vi "mav_msg_decode.vi"(0 "mav_connection_in":T11, 1 "mav_msg":T25, 3 "error in":errorcluster) -> (7 "mav_connection_out":T10, 10 "error out":errorcluster)   [LabVIEW 2023]
uses:
  pfd/pfd_global.vi
  mfd/mfd_global.vi
panel:
  out "HEARTBEAT":T1
  out "WIND":T2
  out "SCALED_PRESSURE2":T3
  out "SCALED_IMU3":T4
  out "SCALED_IMU2":T4
  out "MEMINFO":T5
  out "LOCAL_POSITION_NED":T6
  out "EKF_STATUS_REPORT":T7
  out "AHRS2":T8
  out "BATTERY_STATUS":T9
  out "AUTOPILOT_VERSION":T12
  out "VIBRATION":T13
  out "AOA_SSA":cluster{"time_usec":u64, "AOA":sgl, "SSA":sgl}
  out "AHRS3":T14
  out "AHRS":T15
  out "TERRAIN_REPORT":T16
  out "POWER_STATUS":T17
  out "TIMESYNC":T18
  out "STATUSTEXT":T19(array[cluster])
  out "POSITION_TARGET_GLOBAL_INT":T20
  out "PARAM_VALUE":T21
  out "VFR_HUD":T22
  out "RC_CHANNELS":T23
  out "MISSION_CURRENT":T24
  out "NAV_CONTROLLER_OUTPUT":T26
  out "SERVO_OUTPUT_RAW":T27
  out "GLOBAL_POSITION_INT":T28
  out "ATTITUDE":T29
  out "SCALED_PRESSURE":T3
  out "RAW_IMU":T30
  out "GPS_RAW_INT":T31
  out "SYSTEM_TIME":T32
  out "SYS_STATUS":T33
  out "Message":u32[](array[numeric])
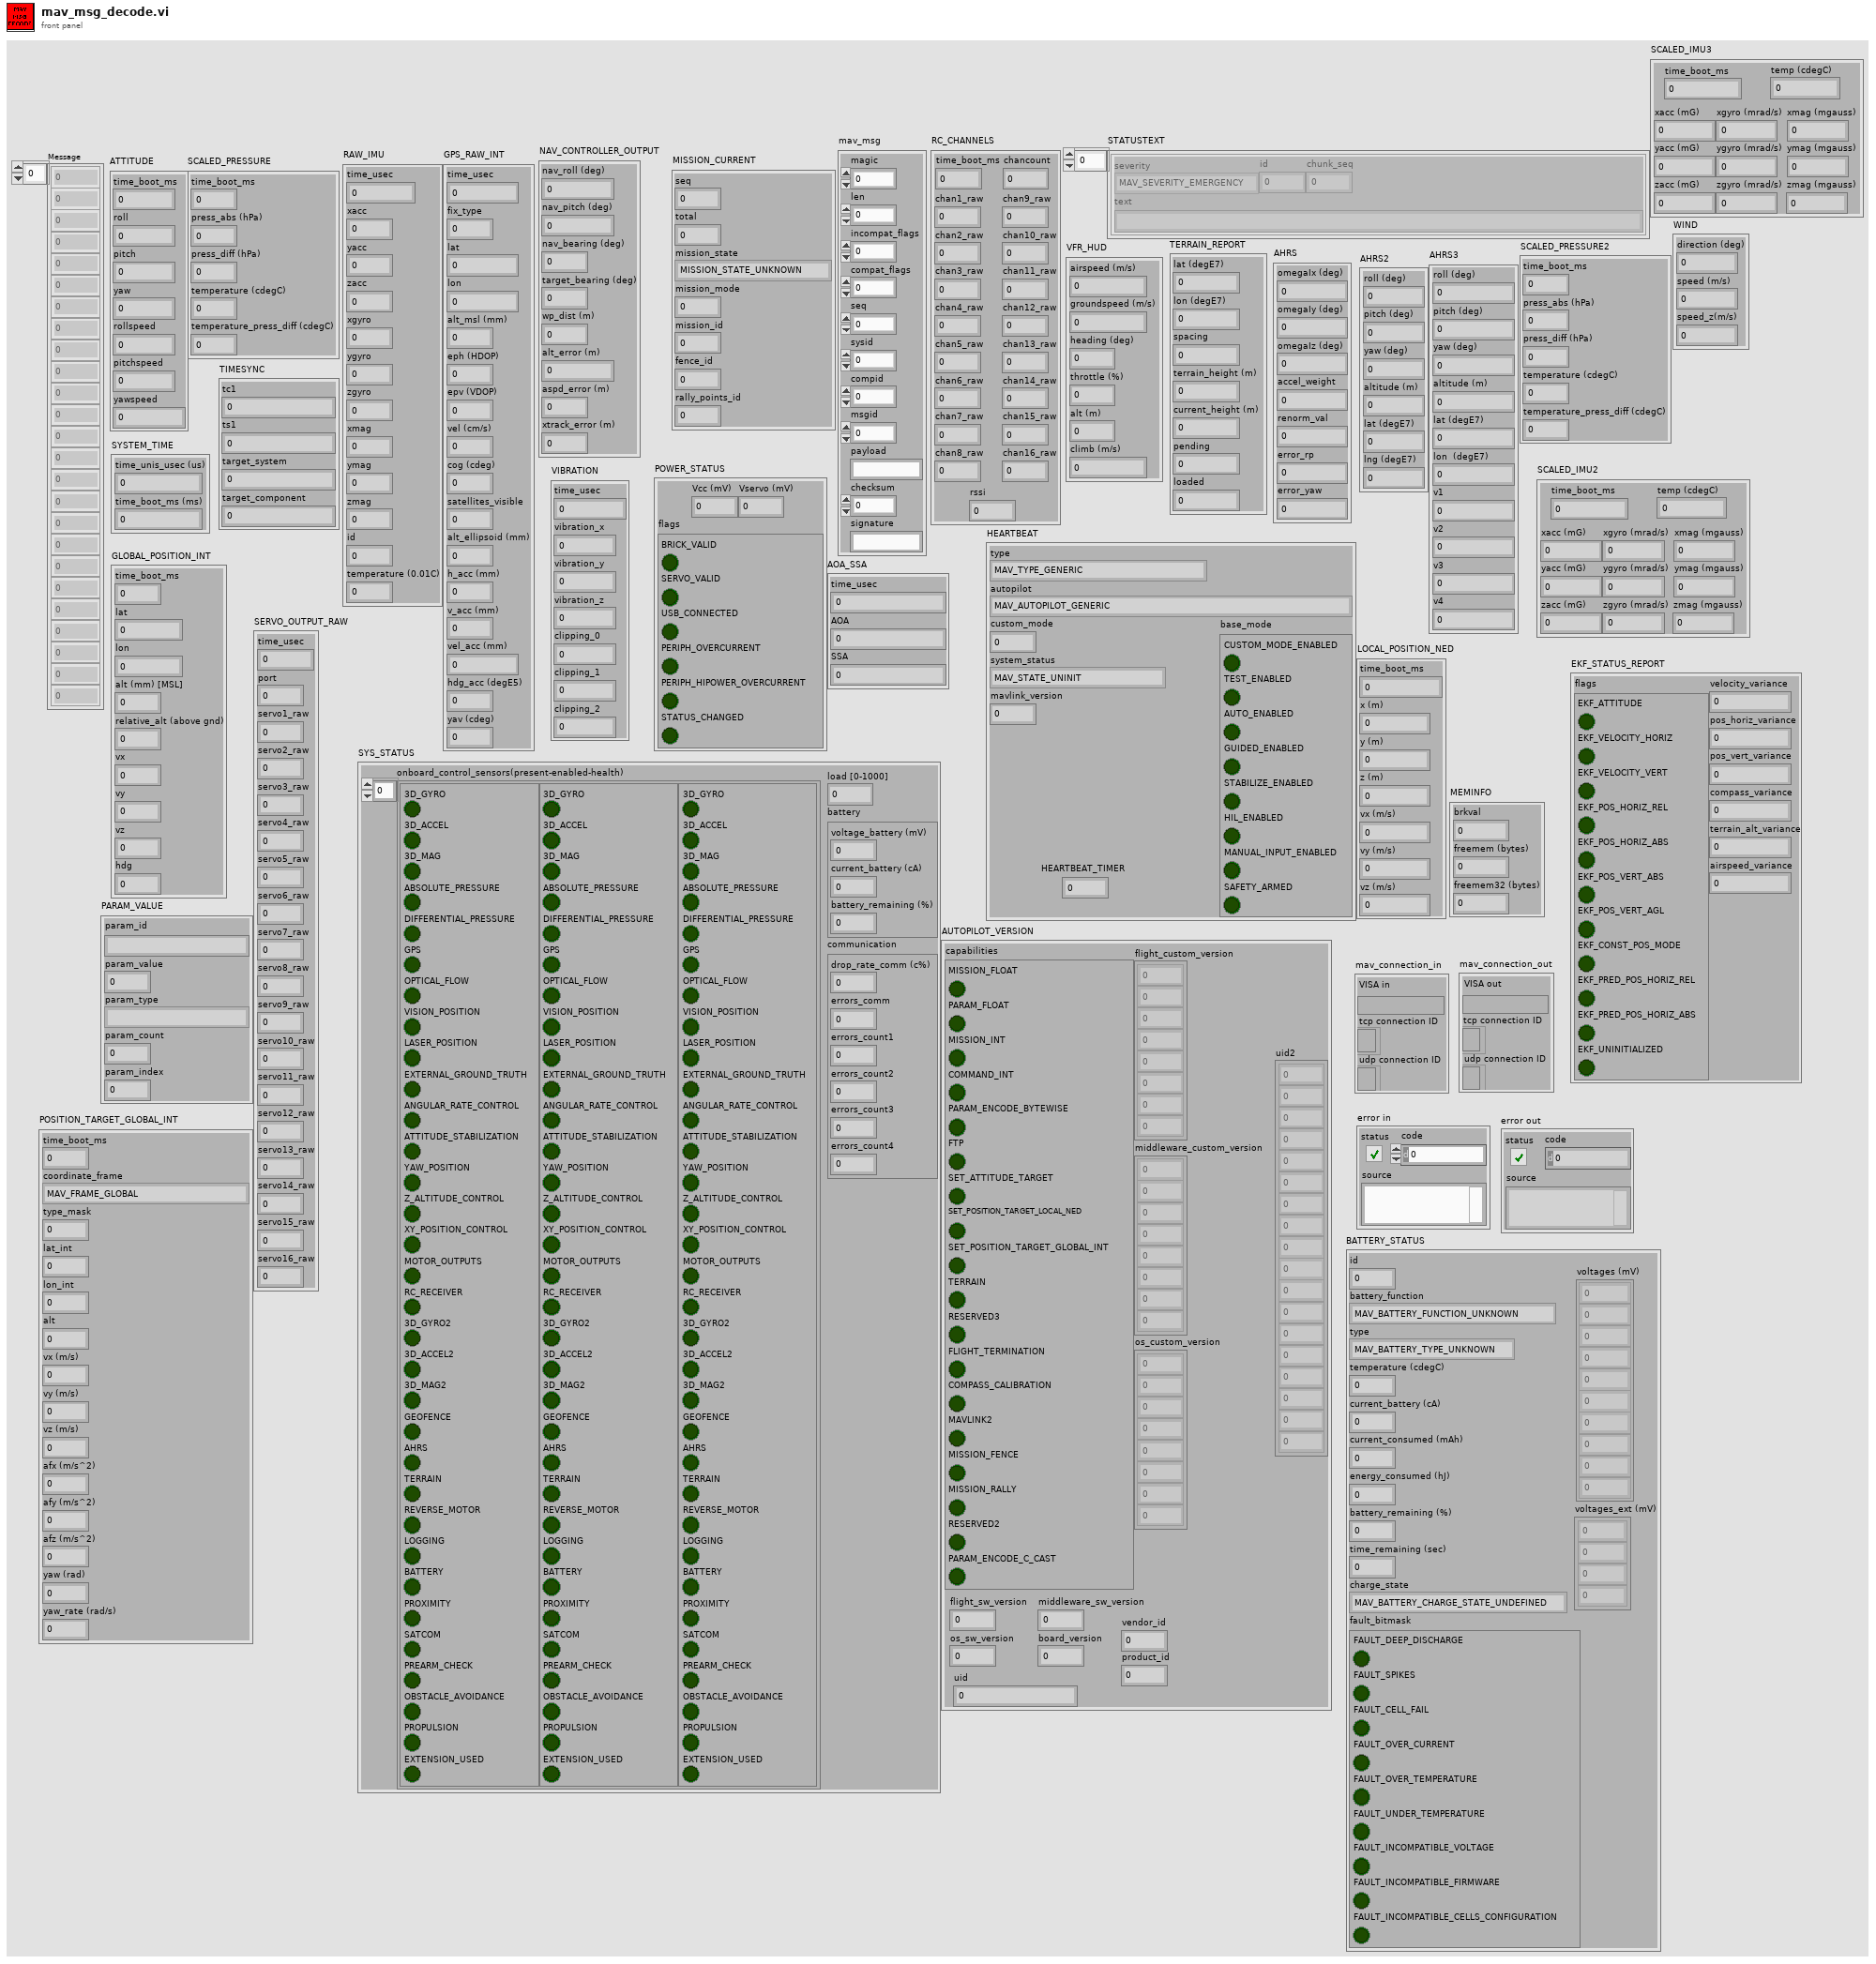
[diagram p1: front panel]
types:
  T1 = cluster{"type":enum8{"MAV_TYPE_GENERIC", "MAV_TYPE_FIXED_WING", "MAV_TYPE_QUADROTOR", "MAV_TYPE_COAXIAL", "MAV_TYPE_HELICOPTER", "MAV_TYPE_ANTENNA_TRACKER", "MAV_TYPE_GCS", "MAV_TYPE_AIRSHIP", "MAV_TYPE_FREE_BALLOON", "MAV_TYPE_ROCKET", "MAV_TYPE_GROUND_ROVER", "MAV_TYPE_SURFACE_BOAT", "MAV_TYPE_SUBMARINE", "MAV_TYPE_HEXAROTOR", "MAV_TYPE_OCTOROTOR", "MAV_TYPE_TRICOPTER", "MAV_TYPE_FLAPPING_WING", "MAV_TYPE_KITE", "MAV_TYPE_ONBOARD_CONTROLLER", "MAV_TYPE_VTOL_TAILSITTER_DUOROTOR", "MAV_TYPE_VTOL_TAILSITTER_QUADROTOR", "MAV_TYPE_VTOL_TILTROTOR", "MAV_TYPE_VTOL_FIXEDROTOR", "MAV_TYPE_VTOL_TAILSITTER", "MAV_TYPE_VTOL_TILTWING", "MAV_TYPE_VTOL_RESERVED5", "MAV_TYPE_GIMBAL", "MAV_TYPE_ADSB", "MAV_TYPE_PARAFOIL", "MAV_TYPE_DODECAROTOR", "MAV_TYPE_CAMERA", "MAV_TYPE_CHARGING_STATION", "MAV_TYPE_FLARM", "MAV_TYPE_SERVO", "MAV_TYPE_ODID", "MAV_TYPE_DECAROTOR", "MAV_TYPE_BATTERY", "MAV_TYPE_PARACHUTE", "MAV_TYPE_LOG", "MAV_TYPE_OSD", "MAV_TYPE_IMU", "MAV_TYPE_GPS", "MAV_TYPE_WINCH", "MAV_TYPE_GENERIC_MULTIROTOR", "MAV_TYPE_ILLUMINATOR"}, "autopilot":enum8{"MAV_AUTOPILOT_GENERIC", "MAV_AUTOPILOT_RESERVED", "MAV_AUTOPILOT_SLUGS", "MAV_AUTOPILOT_ARDUPILOTMEGA", "MAV_AUTOPILOT_OPENPILOT", "MAV_AUTOPILOT_GENERIC_WAYPOINTS_ONLY", "MAV_AUTOPILOT_GENERIC_WAYPOINTS_AND_SIMPLE_NAVIGATION_ONLY", "MAV_AUTOPILOT_GENERIC_MISSION_FULL", "MAV_AUTOPILOT_INVALID", "MAV_AUTOPILOT_PPZ", "MAV_AUTOPILOT_UDB", "MAV_AUTOPILOT_FP", "MAV_AUTOPILOT_PX4", "MAV_AUTOPILOT_SMACCMPILOT", "MAV_AUTOPILOT_AUTOQUAD", "MAV_AUTOPILOT_ARMAZILA", "MAV_AUTOPILOT_AEROB", "MAV_AUTOPILOT_ASLUAV", "MAV_AUTOPILOT_SMARTAP", "MAV_AUTOPILOT_AIRRAILS", "MAV_AUTOPILOT_REFLEX"}, "custom_mode":u32, "system_status":enum16{"MAV_STATE_UNINIT", "MAV_STATE_BOOT", "MAV_STATE_CALIBRATING", "MAV_STATE_STANDBY", "MAV_STATE_ACTIVE", "MAV_STATE_CRITICAL", "MAV_STATE_EMERGENCY", "MAV_STATE_POWEROFF", "MAV_STATE_FLIGHT_TERMINATION"}, "mavlink_version":u8, "base_mode":cluster{"CUSTOM_MODE_ENABLED":bool, "TEST_ENABLED":bool, "AUTO_ENABLED":bool, "GUIDED_ENABLED":bool, "STABILIZE_ENABLED":bool, "HIL_ENABLED":bool, "MANUAL_INPUT_ENABLED":bool, "SAFETY_ARMED":bool}, "HEARTBEAT_TIMER":u32}
  T2 = cluster{"direction (deg)":sgl, "speed (m/s)":sgl, "speed_z(m/s)":sgl}
  T3 = cluster{"time_boot_ms":u32, "press_abs (hPa)":sgl, "press_diff (hPa)":sgl, "temperature (cdegC)":i16, "temperature_press_diff (cdegC)":i16}
  T4 = cluster{"time_boot_ms":u32, "xacc (mG)":i16, "yacc (mG)":i16, "zacc (mG)":i16, "xgyro (mrad/s)":i16, "ygyro (mrad/s)":i16, "zgyro (mrad/s)":i16, "xmag (mgauss)":i16, "ymag (mgauss)":i16, "zmag (mgauss)":i16, "temp (cdegC)":i16}
  T5 = cluster{"brkval":u16, "freemem (bytes)":u16, "freemem32 (bytes)":u32}
  T6 = cluster{"time_boot_ms":u32, "x (m)":sgl, "y (m)":sgl, "z (m)":sgl, "vx (m/s)":sgl, "vy (m/s)":sgl, "vz (m/s)":sgl}
  T7 = cluster{"flags":cluster{"EKF_ATTITUDE":bool, "EKF_VELOCITY_HORIZ":bool, "EKF_VELOCITY_VERT":bool, "EKF_POS_HORIZ_REL":bool, "EKF_POS_HORIZ_ABS":bool, "EKF_POS_VERT_ABS":bool, "EKF_POS_VERT_AGL":bool, "EKF_CONST_POS_MODE":bool, "EKF_PRED_POS_HORIZ_REL":bool, "EKF_PRED_POS_HORIZ_ABS":bool, "EKF_UNINITIALIZED":bool}, "velocity_variance":sgl, "pos_horiz_variance":sgl, "pos_vert_variance":sgl, "compass_variance":sgl, "terrain_alt_variance":sgl, "airspeed_variance":sgl}
  T8 = cluster{"roll (deg)":sgl, "pitch (deg)":sgl, "yaw (deg)":sgl, "altitude (m)":sgl, "lat (degE7)":i32, "lng (degE7)":i32}
  T9 = cluster{"id":u8, "battery_function":enum8{"MAV_BATTERY_FUNCTION_UNKNOWN", "MAV_BATTERY_FUNCTION_ALL", "MAV_BATTERY_FUNCTION_PROPULSION", "MAV_BATTERY_FUNCTION_AVIONICS", "MAV_BATTERY_FUNCTION_PAYLOAD"}, "type":enum8{"MAV_BATTERY_TYPE_UNKNOWN", "MAV_BATTERY_TYPE_LIPO", "MAV_BATTERY_TYPE_LIFE", "MAV_BATTERY_TYPE_LION", "MAV_BATTERY_TYPE_NIMH"}, "temperature (cdegC)":i16, "voltages (mV)":u16[], "current_battery (cA)":i16, "current_consumed (mAh)":i32, "energy_consumed (hJ)":i32, "battery_remaining (%)":i8, "time_remaining (sec)":i32, "charge_state":enum8{"MAV_BATTERY_CHARGE_STATE_UNDEFINED", "MAV_BATTERY_CHARGE_STATE_OK", "MAV_BATTERY_CHARGE_STATE_LOW", "MAV_BATTERY_CHARGE_STATE_CRITICAL", "MAV_BATTERY_CHARGE_STATE_EMERGENCY", "MAV_BATTERY_CHARGE_STATE_FAILED", "MAV_BATTERY_CHARGE_STATE_UNHEALTHY", "MAV_BATTERY_CHARGE_STATE_CHARGING"}, "voltages_ext (mV)":u16[], "fault_bitmask":cluster{"FAULT_DEEP_DISCHARGE":bool, "FAULT_SPIKES":bool, "FAULT_CELL_FAIL":bool, "FAULT_OVER_CURRENT":bool, "FAULT_OVER_TEMPERATURE":bool, "FAULT_UNDER_TEMPERATURE":bool, "FAULT_INCOMPATIBLE_VOLTAGE":bool, "FAULT_INCOMPATIBLE_FIRMWARE":bool, "FAULT_INCOMPATIBLE_CELLS_CONFIGURATION":bool}}
  T10 = cluster{"VISA out":refnum<visa-resource-name>, "tcp connection ID":refnum<k5>, "udp connection ID":refnum<k16>}
  T11 = cluster{"VISA in":refnum<visa-resource-name>, "tcp connection ID":refnum<k5>, "udp connection ID":refnum<k16>}
  T12 = cluster{"flight_sw_version":u32, "middleware_sw_version":u32, "os_sw_version":u32, "board_version":u32, "capabilities":cluster{"MISSION_FLOAT":bool, "PARAM_FLOAT":bool, "MISSION_INT":bool, "COMMAND_INT":bool, "PARAM_ENCODE_BYTEWISE":bool, "FTP":bool, "SET_ATTITUDE_TARGET":bool, "SET_POSITION_TARGET_LOCAL_NED":bool, "SET_POSITION_TARGET_GLOBAL_INT":bool, "TERRAIN":bool, "RESERVED3":bool, "FLIGHT_TERMINATION":bool, "COMPASS_CALIBRATION":bool, "MAVLINK2":bool, "MISSION_FENCE":bool, "MISSION_RALLY":bool, "RESERVED2":bool, "PARAM_ENCODE_C_CAST":bool}, "flight_custom_version":u8[], "middleware_custom_version":u8[], "os_custom_version":u8[], "vendor_id":u16, "product_id":u16, "uid":u64, "uid2":u8[]}
  T13 = cluster{"time_usec":u64, "vibration_x":sgl, "vibration_y":sgl, "vibration_z":sgl, "clipping_0":u32, "clipping_1":u32, "clipping_2":u32}
  T14 = cluster{"roll (deg)":sgl, "pitch (deg)":sgl, "yaw (deg)":sgl, "altitude (m)":sgl, "lat (degE7)":i32, "lon  (degE7)":i32, "v1":sgl, "v2":sgl, "v3":sgl, "v4":sgl}
  T15 = cluster{"omegaIx (deg)":sgl, "omegaIy (deg)":sgl, "omegaIz (deg)":sgl, "accel_weight":sgl, "renorm_val":sgl, "error_rp":sgl, "error_yaw":sgl}
  T16 = cluster{"lat (degE7)":i32, "lon (degE7)":i32, "spacing":u16, "terrain_height (m) ":sgl, "current_height (m) ":sgl, "pending":u16, "loaded":u16}
  T17 = cluster{"Vcc (mV)":u16, "Vservo (mV)":u16, "flags":cluster{"BRICK_VALID":bool, "SERVO_VALID":bool, "USB_CONNECTED":bool, "PERIPH_OVERCURRENT":bool, "PERIPH_HIPOWER_OVERCURRENT":bool, "STATUS_CHANGED":bool}}
  T18 = cluster{"tc1":i64, "ts1":i64, "target_system":u8, "target_component":u8}
  T19 = cluster{"severity":enum8{"MAV_SEVERITY_EMERGENCY", "MAV_SEVERITY_ALERT", "MAV_SEVERITY_CRITICAL", "MAV_SEVERITY_ERROR", "MAV_SEVERITY_WARNING", "MAV_SEVERITY_NOTICE", "MAV_SEVERITY_INFO", "MAV_SEVERITY_DEBUG"}, "id":u16, "chunk_seq":u8, "text":string}[]
  T20 = cluster{"time_boot_ms":u32, "coordinate_frame":enum8{"MAV_FRAME_GLOBAL", "MAV_FRAME_LOCAL_NED", "MAV_FRAME_MISSION", "MAV_FRAME_GLOBAL_RELATIVE_ALT", "MAV_FRAME_LOCAL_ENU", "MAV_FRAME_GLOBAL_INT", "MAV_FRAME_GLOBAL_RELATIVE_ALT_INT", "MAV_FRAME_LOCAL_OFFSET_NED", "MAV_FRAME_BODY_NED", "MAV_FRAME_BODY_OFFSET_NED", "MAV_FRAME_GLOBAL_TERRAIN_ALT", "MAV_FRAME_GLOBAL_TERRAIN_ALT_INT", "MAV_FRAME_BODY_FRD", "MAV_FRAME_RESERVED_13", "MAV_FRAME_RESERVED_14", "MAV_FRAME_RESERVED_15", "MAV_FRAME_RESERVED_16", "MAV_FRAME_RESERVED_17", "MAV_FRAME_RESERVED_18", "MAV_FRAME_RESERVED_19", "MAV_FRAME_LOCAL_FRD", "MAV_FRAME_LOCAL_FLU"}, "type_mask":u16, "lat_int":i32, "lon_int":i32, "alt":sgl, "vx (m/s)":sgl, "vy (m/s)":sgl, "vz (m/s)":sgl, "afx (m/s^2)":sgl, "afy (m/s^2)":sgl, "afz (m/s^2)":sgl, "yaw (rad)":sgl, "yaw_rate (rad/s)":sgl}
  T21 = cluster{"param_id":string, "param_value":sgl, "param_type":enum16{"", "MAV_PARAM_TYPE_UINT8", "MAV_PARAM_TYPE_INT8", "MAV_PARAM_TYPE_UINT16", "MAV_PARAM_TYPE_INT16", "MAV_PARAM_TYPE_UINT32", "MAV_PARAM_TYPE_INT32", "MAV_PARAM_TYPE_UINT64", "MAV_PARAM_TYPE_INT64", "MAV_PARAM_TYPE_REAL32", "MAV_PARAM_TYPE_REAL64"}, "param_count":u16, "param_index":u16}
  T22 = cluster{"airspeed (m/s)":sgl, "groundspeed (m/s)":sgl, "heading (deg) ":i16, "throttle (%) ":u16, "alt (m)":sgl, "climb (m/s)":sgl}
  T23 = cluster{"time_boot_ms":u32, "chancount":u8, "chan1_raw":u16, "chan2_raw":u16, "chan3_raw":u16, "chan4_raw":u16, "chan5_raw":u16, "chan6_raw":u16, "chan7_raw":u16, "chan8_raw":u16, "chan9_raw":u16, "chan10_raw":u16, "chan11_raw":u16, "chan12_raw":u16, "chan13_raw":u16, "chan14_raw":u16, "chan15_raw":u16, "chan16_raw":u16, "rssi":u8}
  T24 = cluster{"seq":u16, "total":u16, "mission_state":enum8{"MISSION_STATE_UNKNOWN", "MISSION_STATE_NO_MISSION", "MISSION_STATE_NOT_STARTED", "MISSION_STATE_ACTIVE", "MISSION_STATE_PAUSED", "MISSION_STATE_COMPLETE"}, "mission_mode":u8, "mission_id":u32, "fence_id":u32, "rally_points_id":u32}
  T25 = cluster{"len":u8, "incompat_flags":u8, "compat_flags":u8, "seq":u8, "sysid":u8, "compid":u8, "msgid":u32, "magic":u8, "payload":string, "checksum":u16, "signature":string}
  T26 = cluster{"nav_roll (deg)":sgl, "nav_pitch (deg)":sgl, "nav_bearing (deg)":i16, "target_bearing (deg)":i16, "wp_dist (m)":u16, "alt_error (m)":sgl, "aspd_error (m)":sgl, "xtrack_error (m)":sgl}
  T27 = cluster{"time_usec":u32, "port":u8, "servo1_raw":u16, "servo2_raw":u16, "servo3_raw":u16, "servo4_raw":u16, "servo5_raw":u16, "servo6_raw":u16, "servo7_raw":u16, "servo8_raw":u16, "servo9_raw":u16, "servo10_raw":u16, "servo11_raw":u16, "servo12_raw":u16, "servo13_raw":u16, "servo14_raw":u16, "servo15_raw":u16, "servo16_raw":u16}
  T28 = cluster{"time_boot_ms":u32, "lat":i32, "lon":i32, "alt (mm) [MSL]":i32, "relative_alt (above gnd)":i32, "vx":i16, "vy":i16, "vz":i16, "hdg":u16}
  T29 = cluster{"time_boot_ms":u32, "roll":sgl, "pitch":sgl, "yaw":sgl, "rollspeed":sgl, "pitchspeed":sgl, "yawspeed":sgl}
  T30 = cluster{"time_usec":u64, "xacc":i16, "yacc":i16, "zacc":i16, "xgyro":i16, "ygyro":i16, "zgyro":i16, "xmag":i16, "ymag":i16, "zmag":i16, "id":u8, "temperature (0.01C)":i16}
  T31 = cluster{"time_usec":u64, "fix_type":u8, "lat":i32, "lon":i32, "alt_msl (mm)":i32, "eph (HDOP)":u16, "epv (VDOP)":u16, "vel (cm/s)":u16, "cog (cdeg)":u16, "satellites_visible":u8, "alt_ellipsoid (mm)":i32, "h_acc (mm)":u32, "v_acc (mm)":u32, "vel_acc (mm)":u32, "hdg_acc (degE5)":u32, "yav (cdeg)":u16}
  T32 = cluster{"time_unis_usec (us)":u64, "time_boot_ms (ms)":u32}
  T33 = cluster{"onboard_control_sensors(present-enabled-health)":cluster{"3D_GYRO":bool, "3D_ACCEL":bool, "3D_MAG":bool, "ABSOLUTE_PRESSURE":bool, "DIFFERENTIAL_PRESSURE":bool, "GPS":bool, "OPTICAL_FLOW":bool, "VISION_POSITION":bool, "LASER_POSITION":bool, "EXTERNAL_GROUND_TRUTH":bool, "ANGULAR_RATE_CONTROL":bool, "ATTITUDE_STABILIZATION":bool, "YAW_POSITION":bool, "Z_ALTITUDE_CONTROL":bool, "XY_POSITION_CONTROL":bool, "MOTOR_OUTPUTS":bool, "RC_RECEIVER":bool, "3D_GYRO2":bool, "3D_ACCEL2":bool, "3D_MAG2":bool, "GEOFENCE":bool, "AHRS":bool, "TERRAIN":bool, "REVERSE_MOTOR":bool, "LOGGING":bool, "BATTERY":bool, "PROXIMITY":bool, "SATCOM":bool, "PREARM_CHECK":bool, "OBSTACLE_AVOIDANCE":bool, "PROPULSION":bool, "EXTENSION_USED":bool}[], "load [0-1000]":u16, "battery":cluster{"voltage_battery (mV)":u16, "current_battery (cA)":i16, "battery_remaining (%)":i8}, "communication":cluster{"drop_rate_comm (c%)":u16, "errors_comm":u16, "errors_count1":u16, "errors_count2":u16, "errors_count3":u16, "errors_count4":u16}}
  T34 = cluster{"chancount":u8, "chan1_raw":u16, "chan2_raw":u16, "chan3_raw":u16, "chan4_raw":u16, "chan5_raw":u16, "chan6_raw":u16, "chan7_raw":u16, "chan8_raw":u16, "chan9_raw":u16, "chan10_raw":u16, "chan11_raw":u16, "chan12_raw":u16, "chan13_raw":u16, "chan14_raw":u16, "chan15_raw":u16, "chan16_raw":u16, "rssi":u8}
  T35 = cluster{"HEARTBEAT":cluster{"type":enum8{"MAV_TYPE_GENERIC", "MAV_TYPE_FIXED_WING", "MAV_TYPE_QUADROTOR", "MAV_TYPE_COAXIAL", "MAV_TYPE_HELICOPTER", "MAV_TYPE_ANTENNA_TRACKER", "MAV_TYPE_GCS", "MAV_TYPE_AIRSHIP", "MAV_TYPE_FREE_BALLOON", "MAV_TYPE_ROCKET", "MAV_TYPE_GROUND_ROVER", "MAV_TYPE_SURFACE_BOAT", "MAV_TYPE_SUBMARINE", "MAV_TYPE_HEXAROTOR", "MAV_TYPE_OCTOROTOR", "MAV_TYPE_TRICOPTER", "MAV_TYPE_FLAPPING_WING", "MAV_TYPE_KITE", "MAV_TYPE_ONBOARD_CONTROLLER", "MAV_TYPE_VTOL_TAILSITTER_DUOROTOR", "MAV_TYPE_VTOL_TAILSITTER_QUADROTOR", "MAV_TYPE_VTOL_TILTROTOR", "MAV_TYPE_VTOL_FIXEDROTOR", "MAV_TYPE_VTOL_TAILSITTER", "MAV_TYPE_VTOL_TILTWING", "MAV_TYPE_VTOL_RESERVED5", "MAV_TYPE_GIMBAL", "MAV_TYPE_ADSB", "MAV_TYPE_PARAFOIL", "MAV_TYPE_DODECAROTOR", "MAV_TYPE_CAMERA", "MAV_TYPE_CHARGING_STATION", "MAV_TYPE_FLARM", "MAV_TYPE_SERVO", "MAV_TYPE_ODID", "MAV_TYPE_DECAROTOR", "MAV_TYPE_BATTERY", "MAV_TYPE_PARACHUTE", "MAV_TYPE_LOG", "MAV_TYPE_OSD", "MAV_TYPE_IMU", "MAV_TYPE_GPS", "MAV_TYPE_WINCH", "MAV_TYPE_GENERIC_MULTIROTOR", "MAV_TYPE_ILLUMINATOR"}, "autopilot":enum8{"MAV_AUTOPILOT_GENERIC", "MAV_AUTOPILOT_RESERVED", "MAV_AUTOPILOT_SLUGS", "MAV_AUTOPILOT_ARDUPILOTMEGA", "MAV_AUTOPILOT_OPENPILOT", "MAV_AUTOPILOT_GENERIC_WAYPOINTS_ONLY", "MAV_AUTOPILOT_GENERIC_WAYPOINTS_AND_SIMPLE_NAVIGATION_ONLY", "MAV_AUTOPILOT_GENERIC_MISSION_FULL", "MAV_AUTOPILOT_INVALID", "MAV_AUTOPILOT_PPZ", "MAV_AUTOPILOT_UDB", "MAV_AUTOPILOT_FP", "MAV_AUTOPILOT_PX4", "MAV_AUTOPILOT_SMACCMPILOT", "MAV_AUTOPILOT_AUTOQUAD", "MAV_AUTOPILOT_ARMAZILA", "MAV_AUTOPILOT_AEROB", "MAV_AUTOPILOT_ASLUAV", "MAV_AUTOPILOT_SMARTAP", "MAV_AUTOPILOT_AIRRAILS", "MAV_AUTOPILOT_REFLEX"}, "custom_mode":u32, "system_status":enum16{"MAV_STATE_UNINIT", "MAV_STATE_BOOT", "MAV_STATE_CALIBRATING", "MAV_STATE_STANDBY", "MAV_STATE_ACTIVE", "MAV_STATE_CRITICAL", "MAV_STATE_EMERGENCY", "MAV_STATE_POWEROFF", "MAV_STATE_FLIGHT_TERMINATION"}, "mavlink_version":u8, "base_mode":cluster{"CUSTOM_MODE_ENABLED":bool, "TEST_ENABLED":bool, "AUTO_ENABLED":bool, "GUIDED_ENABLED":bool, "STABILIZE_ENABLED":bool, "HIL_ENABLED":bool, "MANUAL_INPUT_ENABLED":bool, "SAFETY_ARMED":bool}, "HEARTBEAT_TIMER":u32}, "Batt Stats":cluster{"Active":bool, "State":bool}, "Sat Stats":cluster{"Active":bool, "State":bool}, "Radio Stats":cluster{"Active":bool, "State":bool}, "Sensor Stats":cluster{"Active":bool, "State":bool}}
  T36 = cluster{"3D_GYRO":bool, "3D_ACCEL":bool, "3D_MAG":bool, "ABSOLUTE_PRESSURE":bool, "DIFFERENTIAL_PRESSURE":bool, "GPS":bool, "OPTICAL_FLOW":bool, "VISION_POSITION":bool, "LASER_POSITION":bool, "EXTERNAL_GROUND_TRUTH":bool, "ANGULAR_RATE_CONTROL":bool, "ATTITUDE_STABILIZATION":bool, "YAW_POSITION":bool, "Z_ALTITUDE_CONTROL":bool, "XY_POSITION_CONTROL":bool, "MOTOR_OUTPUTS":bool, "RC_RECEIVER":bool, "3D_GYRO2":bool, "3D_ACCEL2":bool, "3D_MAG2":bool, "GEOFENCE":bool, "AHRS":bool, "TERRAIN":bool, "REVERSE_MOTOR":bool, "LOGGING":bool, "BATTERY":bool, "PROXIMITY":bool, "SATCOM":bool, "PREARM_CHECK":bool, "OBSTACLE_AVOIDANCE":bool, "PROPULSION":bool, "EXTENSION_USED":bool}[]
  T37 = cluster{"voltage_battery (mV)":u16, "current_battery (cA)":i16, "battery_remaining (%)":i8}
  T38 = cluster{"3D_GYRO":bool, "3D_ACCEL":bool, "3D_MAG":bool, "ABSOLUTE_PRESSURE":bool, "DIFFERENTIAL_PRESSURE":bool, "GPS":bool, "OPTICAL_FLOW":bool, "VISION_POSITION":bool, "LASER_POSITION":bool, "EXTERNAL_GROUND_TRUTH":bool, "ANGULAR_RATE_CONTROL":bool, "ATTITUDE_STABILIZATION":bool, "YAW_POSITION":bool, "Z_ALTITUDE_CONTROL":bool, "XY_POSITION_CONTROL":bool, "MOTOR_OUTPUTS":bool, "RC_RECEIVER":bool, "3D_GYRO2":bool, "3D_ACCEL2":bool, "3D_MAG2":bool, "GEOFENCE":bool, "AHRS":bool, "TERRAIN":bool, "REVERSE_MOTOR":bool, "LOGGING":bool, "BATTERY":bool, "PROXIMITY":bool, "SATCOM":bool, "PREARM_CHECK":bool, "OBSTACLE_AVOIDANCE":bool, "PROPULSION":bool, "EXTENSION_USED":bool}
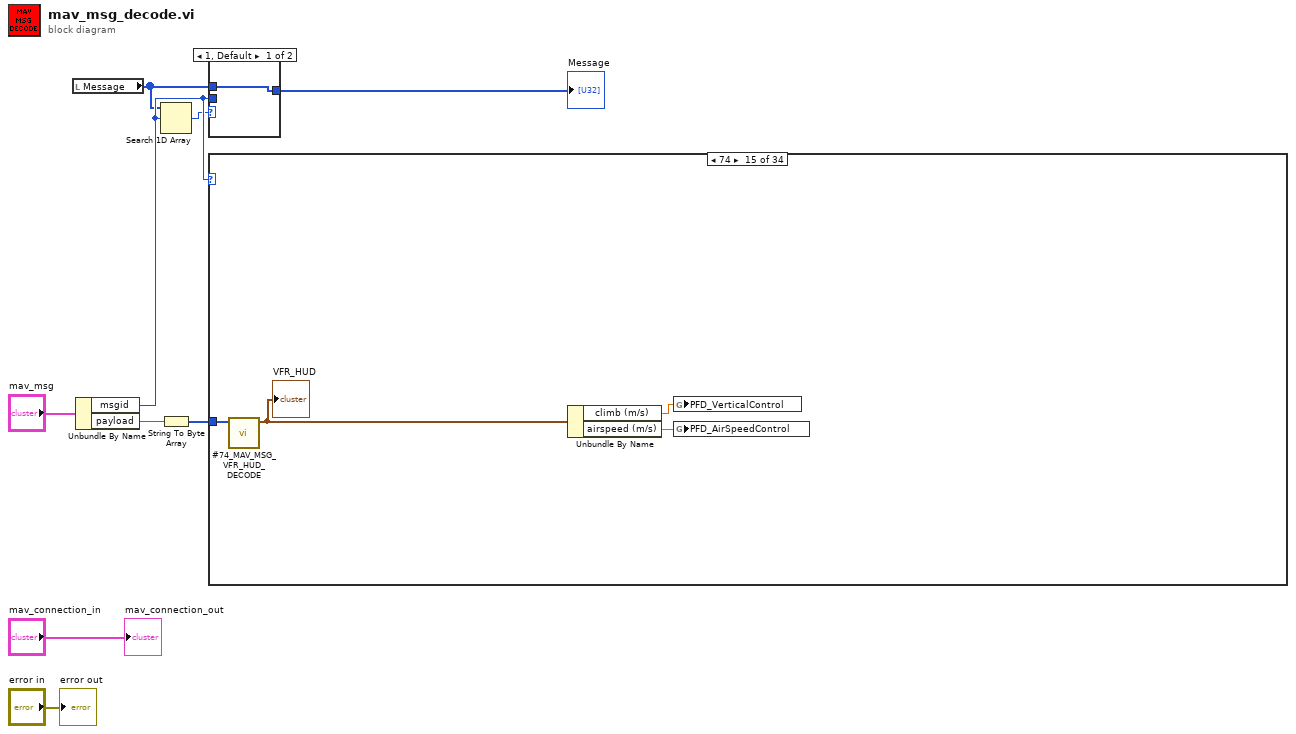
[diagram p0: block diagram]
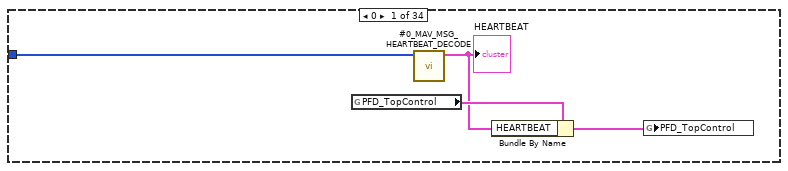
[diagram p2: hidden frame]
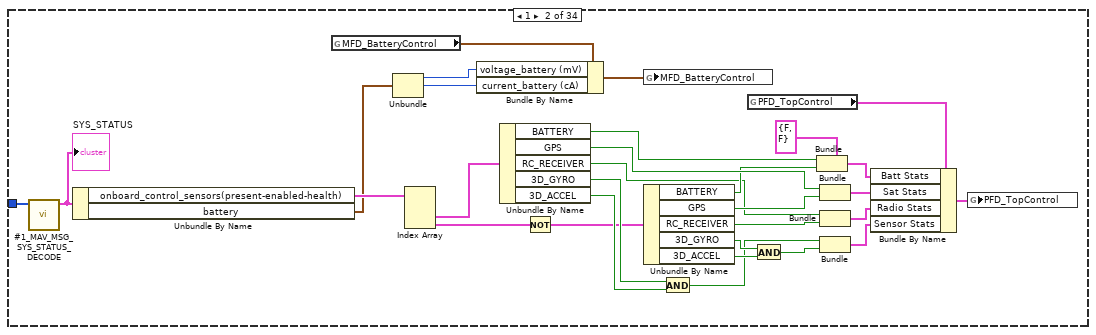
[diagram p3: hidden frame]
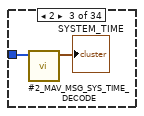
[diagram p4: hidden frame]
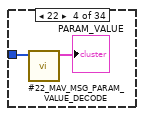
[diagram p5: hidden frame]
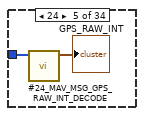
[diagram p6: hidden frame]
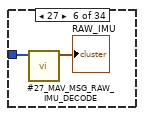
[diagram p7: hidden frame]
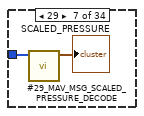
[diagram p8: hidden frame]
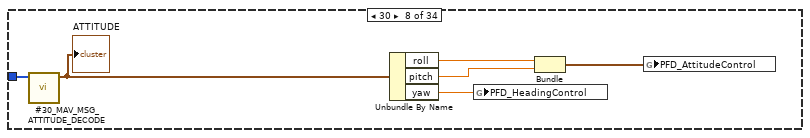
[diagram p9: hidden frame]
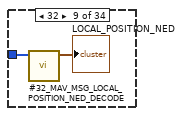
[diagram p10: hidden frame]
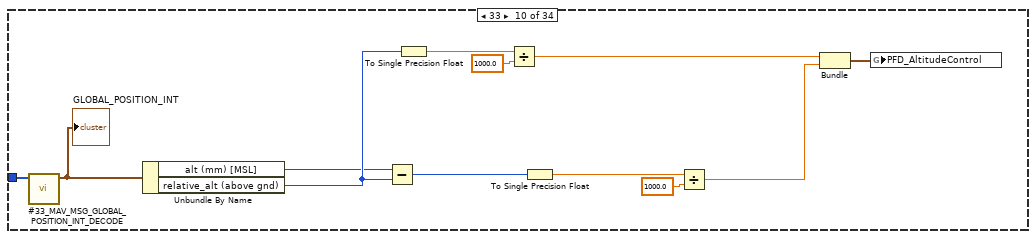
[diagram p11: hidden frame]
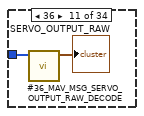
[diagram p12: hidden frame]
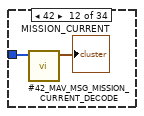
[diagram p13: hidden frame]
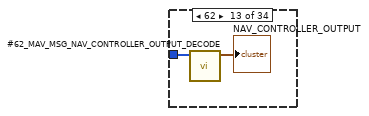
[diagram p14: hidden frame]
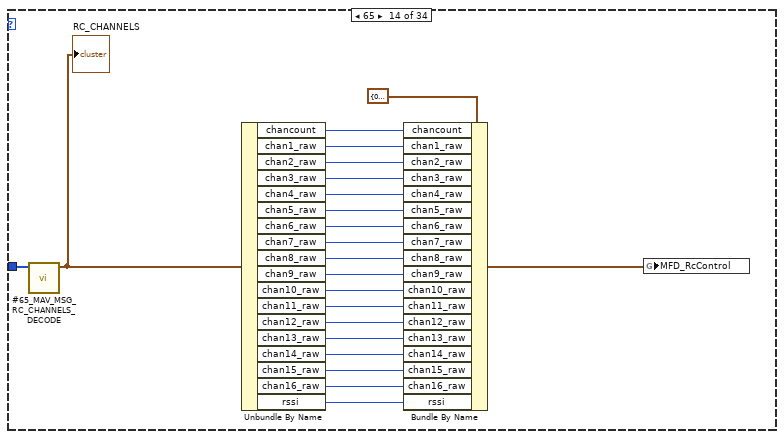
[diagram p15: hidden frame]
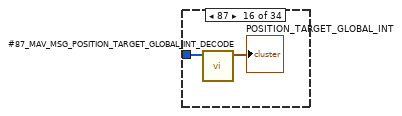
[diagram p16: hidden frame]
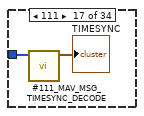
[diagram p17: hidden frame]
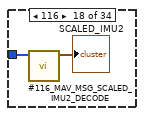
[diagram p18: hidden frame]
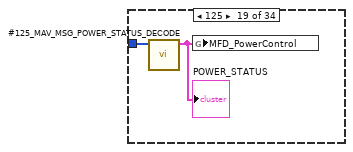
[diagram p19: hidden frame]
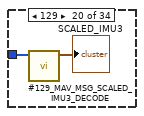
[diagram p20: hidden frame]
diagram:
  n1 = local read "Message"() -> (w3:u32[])
  n2 = Unbundle By Name("mav_msg") -> ("msgid"=w7:u32, "payload"=w8:string)
  n3 = Search 1D Array(1D array=w3, element=w7) -> (index of element=w6:i32)  [unwired: 1 in]
  n4 = String To Byte Array(string=w8) -> (unsigned byte array=w5:u8[])
  n5 = case shown="1, Default" w6 {
    tunnel: w3 -> [w10 w13]
    tunnel: [w10 w12] -> w4
    tunnel: w7 -> [_ w11]
    frame 1, Default {
    }
    frame -1 {
      n6 = Build Array (concatenate)(w13, w11) -> (w12:u32[])
    }
  }
  "Message" <- w4
  n7 = case shown="74" w7 {
    tunnel: w5 -> [w17 w47 w49 w51 w53 w55 w57 w63 w65 w77 w79 w81 w83 w105 w109 w111 w113 w115 w117 w119 w121 w123 w128 w130 w132 w134 w136 w138 w140 w142 w144 w146 _ w148]
    frame 0 {
      n8 = global read "pfd_global.vi" "PFD_TopControl"() -> (w16:T35)
      n9 = call "#0_MAV_MSG_HEARTBEAT_DECODE.vi"("mavlink_payload"=w17) -> ("HEARTBEAT"=w14:T1)  [unwired: 10 in]
      "HEARTBEAT" <- w14
      n10 = Bundle By Name(cluster=w16, "HEARTBEAT"=w14) -> (w15:T35)
      n11 = global write "pfd_global.vi" "PFD_TopControl"(w15) -> ()
    }
    frame 1 {
      n12 = call "#1_MAV_MSG_SYS_STATUS_DECODE.vi"("mavlink_payload"=w47) -> ("SYS_STATUS"=w45:T33)  [unwired: 10 in]
      "SYS_STATUS" <- w45
      n13 = Unbundle By Name(w45) -> ("onboard_control_sensors(present-enabled-health)"=w44:T36, "battery"=w22:T37)
      n14 = global read "mfd_global.vi" "MFD_BatteryControl"() -> (w21:T37)
      n15 = Unbundle(w22) -> ("voltage_battery (mV)"=w19:u16, "current_battery (cA)"=w18:i16)  [unwired: 1 out]
      n16 = Index Array(array=w44) -> (element #2=w43:T38, element #3=w24:T38)  [unwired: 3 in, 1 out]
      n17 = Bundle By Name(cluster=w21, "voltage_battery (mV)"=w19, "current_battery (cA)"=w18) -> (w20:T37)
      n18 = Unbundle By Name(w43) -> ("BATTERY"=w35:bool, "GPS"=w34:bool, "RC_RECEIVER"=w30:bool, "3D_GYRO"=w41:bool, "3D_ACCEL"=w40:bool)
      n19 = Not(x=w24) -> (.not. x?=w23:T38)
      n20 = global write "mfd_global.vi" "MFD_BatteryControl"(w20) -> ()
      n21 = Unbundle By Name(w23) -> ("BATTERY"=w32:bool, "GPS"=w33:bool, "RC_RECEIVER"=w29:bool, "3D_GYRO"=w39:bool, "3D_ACCEL"=w38:bool)
      n22 = And(x=w41, y=w40) -> (x .and. y?=w26:bool)
      n23 = global read "pfd_global.vi" "PFD_TopControl"() -> (w46:T35)
      n24 = And(x=w39, y=w38) -> (x .and. y?=w27:bool)
      n25 = Bundle(cluster=cluster{"Active":bool, "State":bool} {"Active"=FALSE, "State"=FALSE} ("Batt Stats"), "Active"=w35, "State"=w32) -> (w36:cluster{"Active":bool, "State":bool})
      n26 = Bundle("GPS"=w34, "GPS"=w33) -> (w31:cluster{"GPS":bool, "GPS":bool})  [unwired: 1 in]
      n27 = Bundle("RC_RECEIVER"=w30, "RC_RECEIVER"=w29) -> (w28:cluster{"RC_RECEIVER":bool, "RC_RECEIVER":bool})  [unwired: 1 in]
      n28 = Bundle(w26, w27) -> (w25:cluster{bool, bool})  [unwired: 1 in]
      n29 = Bundle By Name(cluster=w46, "Batt Stats"=w36, "Sat Stats"=w31, "Radio Stats"=w28, "Sensor Stats"=w25) -> (w42:T35)
      n30 = global write "pfd_global.vi" "PFD_TopControl"(w42) -> ()
    }
    frame 2 {
      n31 = call "#2_MAV_MSG_SYS_TIME_DECODE.vi"("mavlink_payload"=w49) -> ("SYSTEM_TIME"=→"SYSTEM_TIME":T32)  [unwired: 10 in]
    }
    frame 22 {
      n32 = call "#22_MAV_MSG_PARAM_VALUE_DECODE.vi"("mavlink_payload"=w51) -> ("PARAM_VALUE"=→"PARAM_VALUE":T21)  [unwired: 10 in]
    }
    frame 24 {
      n33 = call "#24_MAV_MSG_GPS_RAW_INT_DECODE.vi"("mavlink_payload"=w53) -> ("GPS_RAW_INT"=→"GPS_RAW_INT":T31)  [unwired: 10 in]
    }
    frame 27 {
      n34 = call "#27_MAV_MSG_RAW_IMU_DECODE.vi"("mavlink_payload"=w55) -> ("RAW_IMU"=→"RAW_IMU":T30)  [unwired: 10 in]
    }
    frame 29 {
      n35 = call "#29_MAV_MSG_SCALED_PRESSURE_DECODE.vi"("mavlink_payload"=w57) -> ("SCALED_PRESSURE"=→"SCALED_PRESSURE":T3)  [unwired: 10 in]
    }
    frame 30 {
      n36 = call "#30_MAV_MSG_ATTITUDE_DECODE.vi"("mavlink_payload"=w63) -> ("ATTITUDE"=w61:T29)  [unwired: 10 in]
      "ATTITUDE" <- w61
      n37 = Unbundle By Name(w61) -> ("roll"=w59:sgl, "pitch"=w60:sgl, "yaw"=w58:sgl)
      n38 = global write "pfd_global.vi" "PFD_HeadingControl"(w58) -> ()
      n39 = Bundle("roll"=w59, "pitch"=w60) -> (w62:cluster{"roll":sgl, "pitch":sgl})  [unwired: 1 in]
      n40 = global write "pfd_global.vi" "PFD_AttitudeControl"(w62) -> ()
    }
    frame 32 {
      n41 = call "#32_MAV_MSG_LOCAL_POSITION_NED_DECODE.vi"("mavlink_payload"=w65) -> ("LOCAL_POSITION_NED"=→"LOCAL_POSITION_NED":T6)  [unwired: 10 in]
    }
    frame 33 {
      n42 = call "#33_MAV_MSG_GLOBAL_POSITION_INT_DECODE.vi"("mavlink_payload"=w77) -> ("GLOBAL_POSITION_INT"=w67:T28)  [unwired: 10 in]
      "GLOBAL_POSITION_INT" <- w67
      n43 = Unbundle By Name(w67) -> ("alt (mm) [MSL]"=w70:i32, "relative_alt (above gnd)"=w71:i32)
      n44 = Subtract(x=w70, y=w71) -> (x-y=w74:i32)
      n45 = To Single Precision Float(number=w71) -> (single precision float=w72:sgl)
      n46 = Divide(x=w72, y=sgl 1000.0) -> (x/y=w73:sgl)
      n47 = To Single Precision Float(number=w74) -> (single precision float=w75:sgl)
      n48 = Divide(x=w75, y=sgl 1000.0) -> (x/y=w76:sgl)
      n49 = Bundle(w73, w76) -> (w66:cluster{sgl, sgl})  [unwired: 1 in]
      n50 = global write "pfd_global.vi" "PFD_AltitudeControl"(w66) -> ()
    }
    frame 36 {
      n51 = call "#36_MAV_MSG_SERVO_OUTPUT_RAW_DECODE.vi"("mavlink_payload"=w79) -> ("SERVO_OUTPUT_RAW"=→"SERVO_OUTPUT_RAW":T27)  [unwired: 10 in]
    }
    frame 42 {
      n52 = call "#42_MAV_MSG_MISSION_CURRENT_DECODE.vi"("mavlink_payload"=w81) -> ("MISSION_CURRENT"=→"MISSION_CURRENT":T24)  [unwired: 10 in]
    }
    frame 62 {
      n53 = call "#62_MAV_MSG_NAV_CONTROLLER_OUTPUT_DECODE.vi"("mavlink_payload"=w83) -> ("NAV_CONTROLLER_OUTPUT"=→"NAV_CONTROLLER_OUTPUT":T26)  [unwired: 10 in]
    }
    frame 65 {
      n54 = call "#65_MAV_MSG_RC_CHANNELS_DECODE.vi"("mavlink_payload"=w105) -> ("RC_CHANNELS"=w102:T23)  [unwired: 10 in]
      "RC_CHANNELS" <- w102
      n55 = Unbundle By Name(w102) -> ("chancount"=w101:u8, "chan1_raw"=w100:u16, "chan2_raw"=w99:u16, "chan3_raw"=w98:u16, "chan4_raw"=w97:u16, "chan5_raw"=w96:u16, "chan6_raw"=w95:u16, "chan7_raw"=w94:u16, "chan8_raw"=w93:u16, "chan9_raw"=w92:u16, "chan10_raw"=w91:u16, "chan11_raw"=w90:u16, "chan12_raw"=w89:u16, "chan13_raw"=w88:u16, "chan14_raw"=w87:u16, "chan15_raw"=w86:u16, "chan16_raw"=w85:u16, "rssi"=w84:u8)
      n56 = Bundle By Name(cluster=T34 {"chancount"=0, "chan1_raw"=0, "chan2_raw"=0, "chan3_raw"=0, "chan4_raw"=0, "chan5_raw"=0, "chan6_raw"=0, "chan7_raw"=0, "chan8_raw"=0, "chan9_raw"=0, "chan10_raw"=0, "chan11_raw"=0, "chan12_raw"=0, "chan13_raw"=0, "chan14_raw"=0, "chan15_raw"=0, "chan16_raw"=0, "rssi"=0} ("MFD_RcControl"), "chancount"=w101, "chan1_raw"=w100, "chan2_raw"=w99, "chan3_raw"=w98, "chan4_raw"=w97, "chan5_raw"=w96, "chan6_raw"=w95, "chan7_raw"=w94, "chan8_raw"=w93, "chan9_raw"=w92, "chan10_raw"=w91, "chan11_raw"=w90, "chan12_raw"=w89, "chan13_raw"=w88, "chan14_raw"=w87, "chan15_raw"=w86, "chan16_raw"=w85, "rssi"=w84) -> (w103:T34)
      n57 = global write "mfd_global.vi" "MFD_RcControl"(w103) -> ()
    }
    frame 74 {
      n58 = call "#74_MAV_MSG_VFR_HUD_DECODE.vi"("mavlink_payload"=w109) -> ("VFR_HUD"=w107:T22)  [unwired: 10 in]
      "VFR_HUD" <- w107
      n59 = Unbundle By Name(w107) -> ("climb (m/s)"=w106:sgl, "airspeed (m/s)"=w108:sgl)
      n60 = global write "PFD_global.vi" "PFD_VerticalControl"(w106) -> ()
      n61 = global write "pfd_global.vi" "PFD_AirSpeedControl"(w108) -> ()
    }
    frame 87 {
      n62 = call "#87_MAV_MSG_POSITION_TARGET_GLOBAL_INT_DECODE.vi"("mavlink_payload"=w111) -> ("POSITION_TARGET_GLOBAL_INT"=→"POSITION_TARGET_GLOBAL_INT":T20)  [unwired: 10 in]
    }
    frame 111 {
      n63 = call "#111_MAV_MSG_TIMESYNC_DECODE.vi"("mavlink_payload"=w113) -> ("TIMESYNC"=→"TIMESYNC":T18)  [unwired: 10 in]
    }
    frame 116 {
      n64 = call "#116_MAV_MSG_SCALED_IMU2_DECODE.vi"("mavlink_payload"=w115) -> ("SCALED_IMU2"=→"SCALED_IMU2":T4)  [unwired: 10 in]
    }
    frame 125 {
      n65 = call "#125_MAV_MSG_POWER_STATUS_DECODE.vi"("mavlink_payload"=w117) -> ("POWER_STATUS"=w116:T17)  [unwired: 10 in]
      "POWER_STATUS" <- w116
      n66 = global write "mfd_global.vi" "MFD_PowerControl"(w116) -> ()
    }
    frame 129 {
      n67 = call "#129_MAV_MSG_SCALED_IMU3_DECODE.vi"("mavlink_payload"=w119) -> ("SCALED_IMU3"=→"SCALED_IMU3":T4)  [unwired: 10 in]
    }
    frame 136 {
      n68 = call "#136_MAV_MSG_TERRAIN_REPORT_DECODE.vi"("mavlink_payload"=w121) -> ("TERRAIN_REPORT"=→"TERRAIN_REPORT":T16)  [unwired: 10 in]
    }
    frame 137 {
      n69 = call "#137_MAV_MSG_ID_SCALED_PRESSURE2_DECODE.vi"("mavlink_payload"=w123) -> ("SCALED_PRESSURE2"=→"SCALED_PRESSURE2":T3)  [unwired: 10 in]
    }
    frame 147 {
      n70 = call "#147_MAV_MSG_BATTERY_STATUS_DECODE.vi"("mavlink_payload"=w128) -> ("BATTERY_STATUS"=w127:T9)  [unwired: 10 in]
      "BATTERY_STATUS" <- w127
      n71 = Unbundle By Name(w127) -> ("battery_remaining (%)"=w125:i8)
      n72 = global read "mfd_global.vi" "MFD_BatteryControl"() -> (w126:T37)
      n73 = Bundle By Name(cluster=w126, "battery_remaining (%)"=w125) -> (w124:T37)
      n74 = global write "mfd_global.vi" "MFD_BatteryControl"(w124) -> ()
    }
    frame 148 {
      n75 = call "#148_MAV_MSG_AUTOPILOT_VERSION_DECODE.vi"("mavlink_payload"=w130) -> ("AUTOPILOT_VERSION"=→"AUTOPILOT_VERSION":T12)  [unwired: 10 in]
    }
    frame 152 {
      n76 = call "#152_MAV_MSG_MEMINFO_DECODE.vi"("mavlink_payload"=w132) -> ("MEMINFO"=→"MEMINFO":T5)  [unwired: 10 in]
    }
    frame 163 {
      n77 = call "#163_MAV_MSG_AHRS_DECODE.vi"("mavlink_payload"=w134) -> ("AHRS"=→"AHRS":T15)  [unwired: 10 in]
    }
    frame 168 {
      n78 = call "#168_MAV_MSG_WIND_DECODE.vi"("mavlink_payload"=w136) -> ("WIND"=→"WIND":T2)  [unwired: 10 in]
    }
    frame 178 {
      n79 = call "#178_MAV_MSG_AHRS2_DECODE.vi"("mavlink_payload"=w138) -> ("AHRS2"=→"AHRS2":T8)  [unwired: 10 in]
    }
    frame 182 {
      n80 = call "#182_MAV_MSG_AHRS3_DECODE.vi"("mavlink_payload"=w140) -> ("AHRS3"=→"AHRS3":T14)  [unwired: 10 in]
    }
    frame 193 {
      n81 = call "#193_MAV_MSG_EKF_STATUS_REPORT_DECODE.vi"("mavlink_payload"=w142) -> ("EKF_STATUS_REPORT"=→"EKF_STATUS_REPORT":T7)  [unwired: 10 in]
    }
    frame 241 {
      n82 = call "#241_MAV_MSG_VIBRATION_DECODE.vi"("mavlink_payload"=w144) -> ("VIBRATION"=→"VIBRATION":T13)  [unwired: 10 in]
    }
    frame 253 {
      n83 = call "#253_MAV_MSG_STATUSTEXT_DECODE.vi"("mavlink_payload"=w146) -> ("STATUSTEXT"=w145:T19)  [unwired: 10 in]
      "STATUSTEXT" <- w145
      n84 = global write "mfd_global.vi" "MFD_StatusTextControl"(w145) -> ()
    }
    frame 255, Default {
    }
    frame 11020 {
      n85 = call "#11020_MAV_MSG_AOA_SSA_DECODE.vi"("mavlink_payload"=w148) -> ("AOA_SSA"=→"AOA_SSA":cluster{"time_usec":u64, "AOA":sgl, "SSA":sgl})  [unwired: 10 in]
    }
  }
  "mav_connection_out" <- "mav_connection_in"
  "error out" <- "error in"
